vi "Pre Launch Init.vi"(11 "Modbus in":refnum<class "Modbus.lvclass">) -> (0 "error out":errorcluster, 3 "Modbus out":refnum<class "Modbus.lvclass">)   [LabVIEW 2020, in "Modbus.lvlib" / "Modbus.lvclass"]
doc: "(<B>Filename</B>: Actor Framework.lvlib:Actor.lvclass:Pre Launch Init.vi)\n\nDefines behavior that occurs after the Launch Nested Actor method is invoked but before the actor's Actor Core method begins running.\n\nBy default, this method does nothing. A descendant class may override it to define behavior."
uses:
  Modbus.lvclass
  Modbus.lvclass/Modbus.ctl
  <vilib>/Instr/_visa.llb/VISA Configure Serial Port (Instr).vi
  Sensor/Sensor/Sensor.lvclass
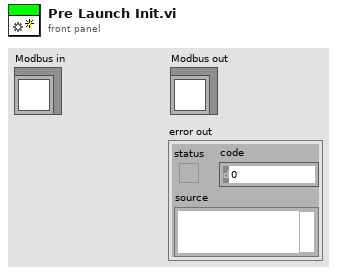
[diagram p1: front panel]
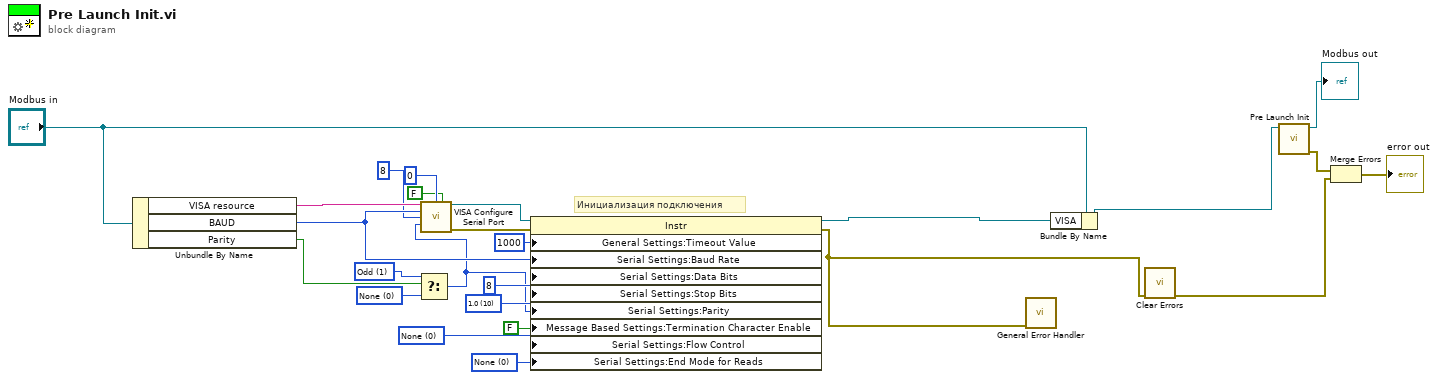
[diagram p0: block diagram]
diagram:
  w13 = u16 1 items=["None", "Odd", "Even", "Mark", "Space"] ("Serial Settings:Parity")
  w15 = u16 0 items=["None", "Odd", "Even", "Mark", "Space"] ("Serial Settings:Parity")
  w23 = u16 0 items=["None", "XON/XOFF", "RTS/CTS", "XON/XOFF & RTS/CTS", "DTR/DSR", "XON/XOFF & DTR/DSR"] ("Serial Settings:Flow Control")
  w20 = u16 0 items=["None", "LastBit", "TermChar"] ("Serial Settings:Serial End Mode for Reads")
  w18 = u16 10 items=["1.0"=10, "1.5"=15, "2.0"=20] ("Serial Settings:Serial Stop Bits")
  # "Инициализация подключения"
  n1 = Unbundle By Name("Modbus in") -> ("VISA resource"=w17:string, "BAUD"=w5:u16, "Parity"=w14:bool)
  n2 = Select(t=w13, s=w14, f=w15) -> (s? t:f=w3:u16)
  n3 = call-poly "VISA Configure Serial Port"("VISA resource name"=w17, "termination char\n(0xA = '\\n' = LF)"=u8 0 ("termination char\n(0xA = '\\n' = LF)"), "Enable Termination\nChar (T)"=FALSE ("Enable Termination\nChar (T)"), "baud rate (9600)"=w5, "data bits (8)"=u16 8, "parity (0:none)"=w3) -> ("VISA resource name out"=w22:refnum<visa-resource-name>, "error out"=w16:errorcluster)  [unwired: 8 in]
  n4 = property class="Instr"(reference=w22, error in=w16, "General Settings:Timeout Value"=u32 1000, "Serial Settings:Baud Rate"=w5, "Serial Settings:Data Bits"=u16 8 ("data bits"), "Serial Settings:Stop Bits"=w18, "Serial Settings:Parity"=w3, "Message Based Settings:Termination Character Enable"=FALSE, "Serial Settings:Flow Control"=w23, "Serial Settings:End Mode for Reads"=w20) -> (reference out=w7:refnum<visa-resource-name>, error out=w6:errorcluster)
  n5 = call <vilib>:"General Error Handler.vi"("error in (no error)"=w6) -> ()  [unwired: 10 in, 5 out]
  n6 = Bundle By Name(cluster="Modbus in", "VISA"=w7) -> (w9:refnum<class "Modbus.lvclass">)
  n7 = call <vilib>:"Clear Errors.vi"("error in (no error)"=w6) -> ("error out"=w8:errorcluster)  [unwired: 5 in, 1 out]
  n8 = call-parent "Pre Launch Init.vi"("Sensor in"=w9) -> ("error out"=w12:errorcluster, "Sensor out"=→"Modbus out":refnum<class "Modbus.lvclass">)  [unwired: 9 in]
  n9 = Merge Errors(w12, w8) -> (→"error out":errorcluster)
